vi "ScopeIntegrateSignal_v2.vi"() -> ()   [LabVIEW 2018]
doc: "This example illustrates how to use autosetup and continuously acquires waveforms from a single channel using the following steps:\n\n1. Specify a valid VISA session. \n2. Specify a channel. \n3. Specify a time-out value for reading waveform.\n4. Run the VI. The graph displays the waveform you acquire."
uses:
  <vilib>/Analysis/baseanly.llb/Mean (DBL).vi
  <instrlib>/Tektronix DPO MSO 2000 4000 Series/Public/Data/Read (Single Waveform).vi
  <vilib>/Waveform/WDTOps.llb/WDT Get Waveform Subset DBL.vi
  <instrlib>/Tektronix DPO MSO 2000 4000 Series/Tektronix DPO MSO 2000 4000 Series.lvlib
  <vilib>/Analysis/NI_AALBase.lvlib
panel:
  in  "Tab Control":enum32{"Page 1", "Page 2"}(tab)
  out "Waveform Graph":waveform(dbl)(graph)={"t0"=timestamp(-0.00019999999999997797 s since 1904-01-01), "dt"=4e-10, "Y"=array[1000000 elements]}
  out "x-y":dbl format="%#_4f"
  in  "thresh":dbl=0.01 format="%_3p"
  out "sig start":dbl=0.0020477815699658703
  out "sig stop":dbl=0.004027303754266211
  out "bkgd start":dbl=0.006484641638225256
  out "bkgd stop":dbl=0.009488054607508532
  out "Numeric":i32
  in  "Maximum Time (10000ms)":u32=10000
  in  "VISA Resource Name":refnum<visa-resource-name>="mdo4034c"
  out "dt":dbl=4e-10
  in  "Acquire":bool=TRUE
  in  "Looping?":bool
  in  "stop":bool
  in  "Channel \n(0: Channel 1)":u16(ring) items=["Channel 1", "Channel 2", "Channel 3", "Channel 4", "Math", "Reference 1", "Reference 2", "Reference 3", "Reference 4"]
  # "(C) 2006 - 2022. National Instruments Corporation. ALL RIGHTS RESERVED."
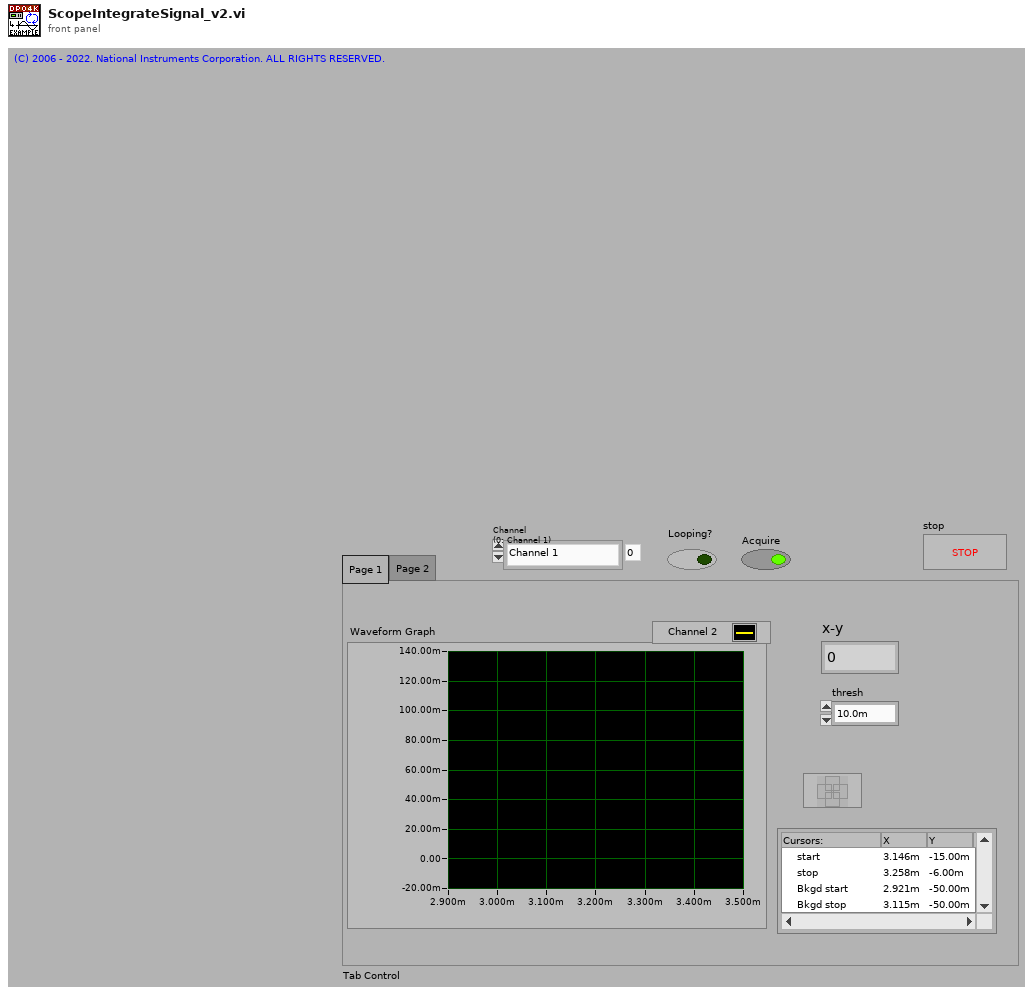
[diagram p1: front panel]
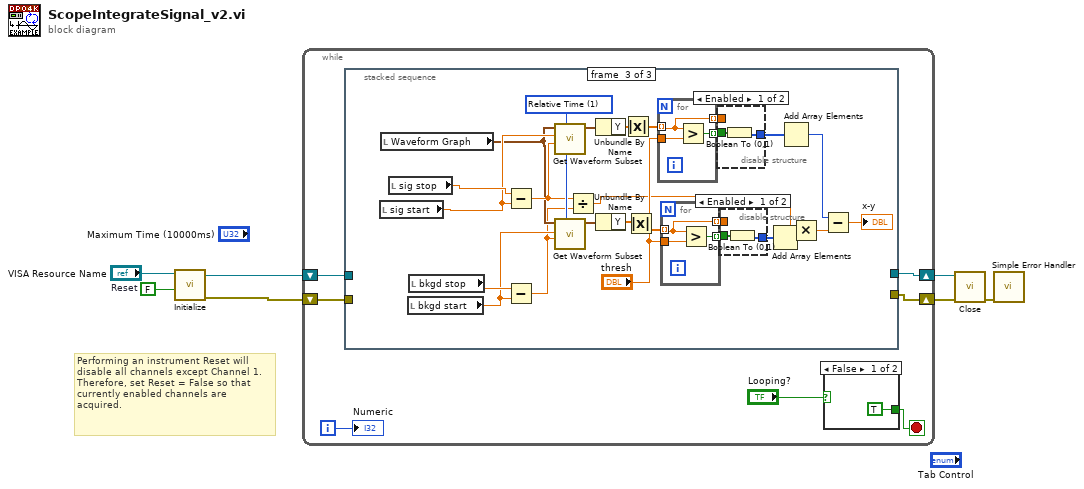
[diagram p0: block diagram]
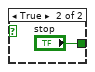
[diagram p2: hidden frame]
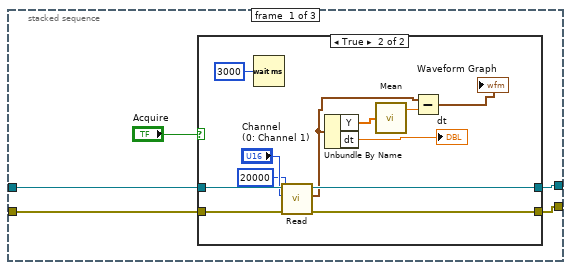
[diagram p3: hidden frame]
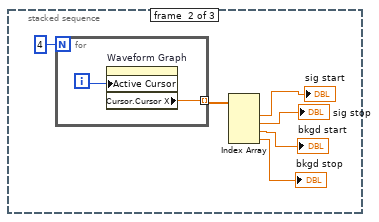
[diagram p5: hidden frame]
diagram:
  w3 = FALSE  # Reset
  # "Performing an instrument Reset will disable all channels except Channel 1. Therefore, set Reset = False so that currently enabled channels are acquired."
  n1 = call <instrlib>:"Initialize.vi"("Reset (True)"=w3, "VISA resource name"="VISA Resource Name") -> ("error out"=w2:errorcluster, "VISA resource name out"=w1:refnum<visa-resource-name>)  [unwired: 8 in]
  n2 = while {
    shift-right: [w8] -> w5
    shift-left: w2 -> [w14]
    shift-right: [w9] -> w6
    shift-left: w1 -> [w13]
    i -> [w10]
    stop <- w11 stop-if-true
    n3 = stacked-sequence {
      tunnel: w13 -> [w21 _ _]
      tunnel: w14 -> [w20 _ _]
      tunnel: [w19 _ _] -> w9
      tunnel: [w18 _ _] -> w8
      frame #0 {
        n4 = case shown="True" "Acquire" {
          tunnel: w21 -> [w23 w35]
          tunnel: w20 -> [w22 w34]
          tunnel: [w23 w32] -> w19
          tunnel: [w22 w31] -> w18
          frame False {
          }
          frame True {
            n5 = Wait (ms)(milliseconds to wait=u32 3000) -> ()  [unwired: 1 out]
            n6 = call-poly <instrlib>:"Read.vi"("error in (no error)"=w34, "Maximum Time (10000ms)"=u32 20000, "Channel (0: Channel 1)"="Channel \n(0: Channel 1)", "VISA resource name"=w35) -> ("error out"=w31:errorcluster, "Waveform Graph"=w26:waveform(dbl), "VISA resource name out"=w32:refnum<visa-resource-name>)  [unwired: 5 in]
            n7 = Unbundle By Name(w26) -> ("Y"=w28:dbl[], "dt"=→"dt":dbl)
            n8 = call-poly <vilib>:"Mean.vi"("X"=w28) -> ("mean"=w27:dbl)  [unwired: 1 out]
            n9 = Subtract(x=w26, y=w27) -> (x-y=→"Waveform Graph":waveform(dbl))
          }
        }
      }
      frame #1 {
        n10 = for {
          N: 4 -> [_]
          tunnel: [w42] -> w40 mode=indexing
          i -> [w43]
          n11 = property on="Waveform Graph" class="WFGraph (strict)"("Active Cursor"=w43) -> ("Cursor.Cursor X"=w42:dbl)  [unwired: 2 in, 2 out]
        }
        n12 = Index Array(array=w40) -> (element #1=→"sig start":dbl, element #2=→"sig stop":dbl, element #3=→"bkgd start":dbl, element #4=→"bkgd stop":dbl)  [unwired: 4 in]
      }
      frame #2 {
        w65 = u16 1 items=["Samples", "Relative Time"] ("start/duration format")
        n13 = local read "sig start"() -> (w66:dbl)
        n14 = local read "Waveform Graph"() -> (w63:waveform(dbl))
        n15 = local read "sig stop"() -> (w67:dbl)
        n16 = local read "bkgd start"() -> (w68:dbl)
        n17 = local read "bkgd stop"() -> (w69:dbl)
        n18 = Subtract(x=w67, y=w66) -> (x-y=w64:dbl)
        n19 = Subtract(x=w69, y=w68) -> (x-y=w62:dbl)
        n20 = call-poly <vilib>:"Get Waveform Subset.vi"("start/duration format"=w65, "duration"=w64, "start samples/time"=w66, "waveform in"=w63) -> ("waveform out"=w61:waveform(dbl))  [unwired: 2 in, 3 out]
        n21 = call-poly <vilib>:"Get Waveform Subset.vi"("start/duration format"=w65, "duration"=w62, "start samples/time"=w68, "waveform in"=w63) -> ("waveform out"=w60:waveform(dbl))  [unwired: 2 in, 3 out]
        n22 = Divide(x=w64, y=w62) -> (x/y=w51:dbl)
        n23 = Unbundle By Name(w61) -> ("Y"=w59:dbl[])
        n24 = Unbundle By Name(w60) -> ("Y"=w54:dbl[])
        n25 = Absolute Value(x=w59) -> (abs(x)=w45:dbl[])
        n26 = Absolute Value(x=w54) -> (abs(x)=w44:dbl[])
        n27 = for {
          tunnel: w45 -> [w79] mode=indexing
          tunnel: "thresh" -> [w81]
          tunnel: [w80] -> w58 mode=indexing
          tunnel: [w79] -> w47 mode=indexing
          n28 = Greater?(x=w79, y=w81) -> (0:w80:bool)
        }
        n29 = for {
          tunnel: w44 -> [w76] mode=indexing
          tunnel: "thresh" -> [w78]
          tunnel: [w77] -> w55 mode=indexing
          tunnel: [w76] -> w46 mode=indexing
          n30 = Greater?(x=w76, y=w78) -> (0:w77:bool)
        }
        n31 = disable-structure shown="Enabled" {
          disable-tunnel: w58 -> [w74 _]
          disable-tunnel: [w73 w75] -> w57
          disable-tunnel: w47 -> [_ w75]
          frame Enabled {
            n32 = Boolean To (0,1)(Boolean=w74) -> (0, 1=w73:i16[])
          }
          frame Disabled {
          }
        }
        n33 = disable-structure shown="Enabled" {
          disable-tunnel: [w71 w72] -> w56
          disable-tunnel: w55 -> [w70 _]
          disable-tunnel: w46 -> [_ w72]
          frame Enabled {
            n34 = Boolean To (0,1)(Boolean=w70) -> (0, 1=w71:i16[])
          }
          frame Disabled {
          }
        }
        n35 = Add Array Elements(numeric array=w56) -> (sum=w52:i16)
        n36 = Add Array Elements(numeric array=w57) -> (sum=w49:i16)
        n37 = Multiply(x=w51, y=w52) -> (x*y=w50:dbl)
        n38 = Subtract(x=w49, y=w50) -> (x-y=→"x-y":dbl)
      }
    }
    n39 = case shown="False" "Looping?" {
      tunnel: [TRUE ("stop") "stop"] -> w11
      frame False {
      }
      frame True {
      }
    }
    "Numeric" <- w10
  }
  n40 = call <instrlib>:"Close.vi"("error in (no error)"=w5, "VISA resource name"=w6) -> ("error out"=w4:errorcluster)  [unwired: 9 in]
  n41 = call <vilib>:"Simple Error Handler.vi"("error in (no error)"=w4) -> ()  [unwired: 4 in, 5 out]
